vi "Table_Script.vi"() -> ()   [LabVIEW 2020]
uses:
  <userlib>/_OpenG.lib/array/array.llb/Index 1D Array Elements (String)__ogtk.vi
  <vilib>/regexp/Match Regular Expression.xnode
  <vilib>/addons/database/NI_Database_API.lvlib
panel:
  in  "Push Mind Script":string
  in  "Update Trigger":string
  in  "Insert Trigger":string
  in  "SELECT Into":string
  out "tables":string[](array[string])
  in  "HMI Script":string
  in  "PLC Tags":string
  in  "OPC Tag":bool
  in  "INSERTED":string
  in  "OPC Tags":string
  in  "Cluster":bool
  in  "Declare":string
  in  "Include Space":bool
  in  "Include Set Bracket":bool=TRUE
  in  "Script Column":string
  in  "Table List":i32[](listbox)
  # "Tag Name,Address,Data Type,Respect Data Type,Client Access,Scan Rate,Scaling,Raw Low,Raw High,Scaled Low,Scaled High,Scaled Data Type,Clamp Low,Clamp High,Eng Units,Description,Negate Value"
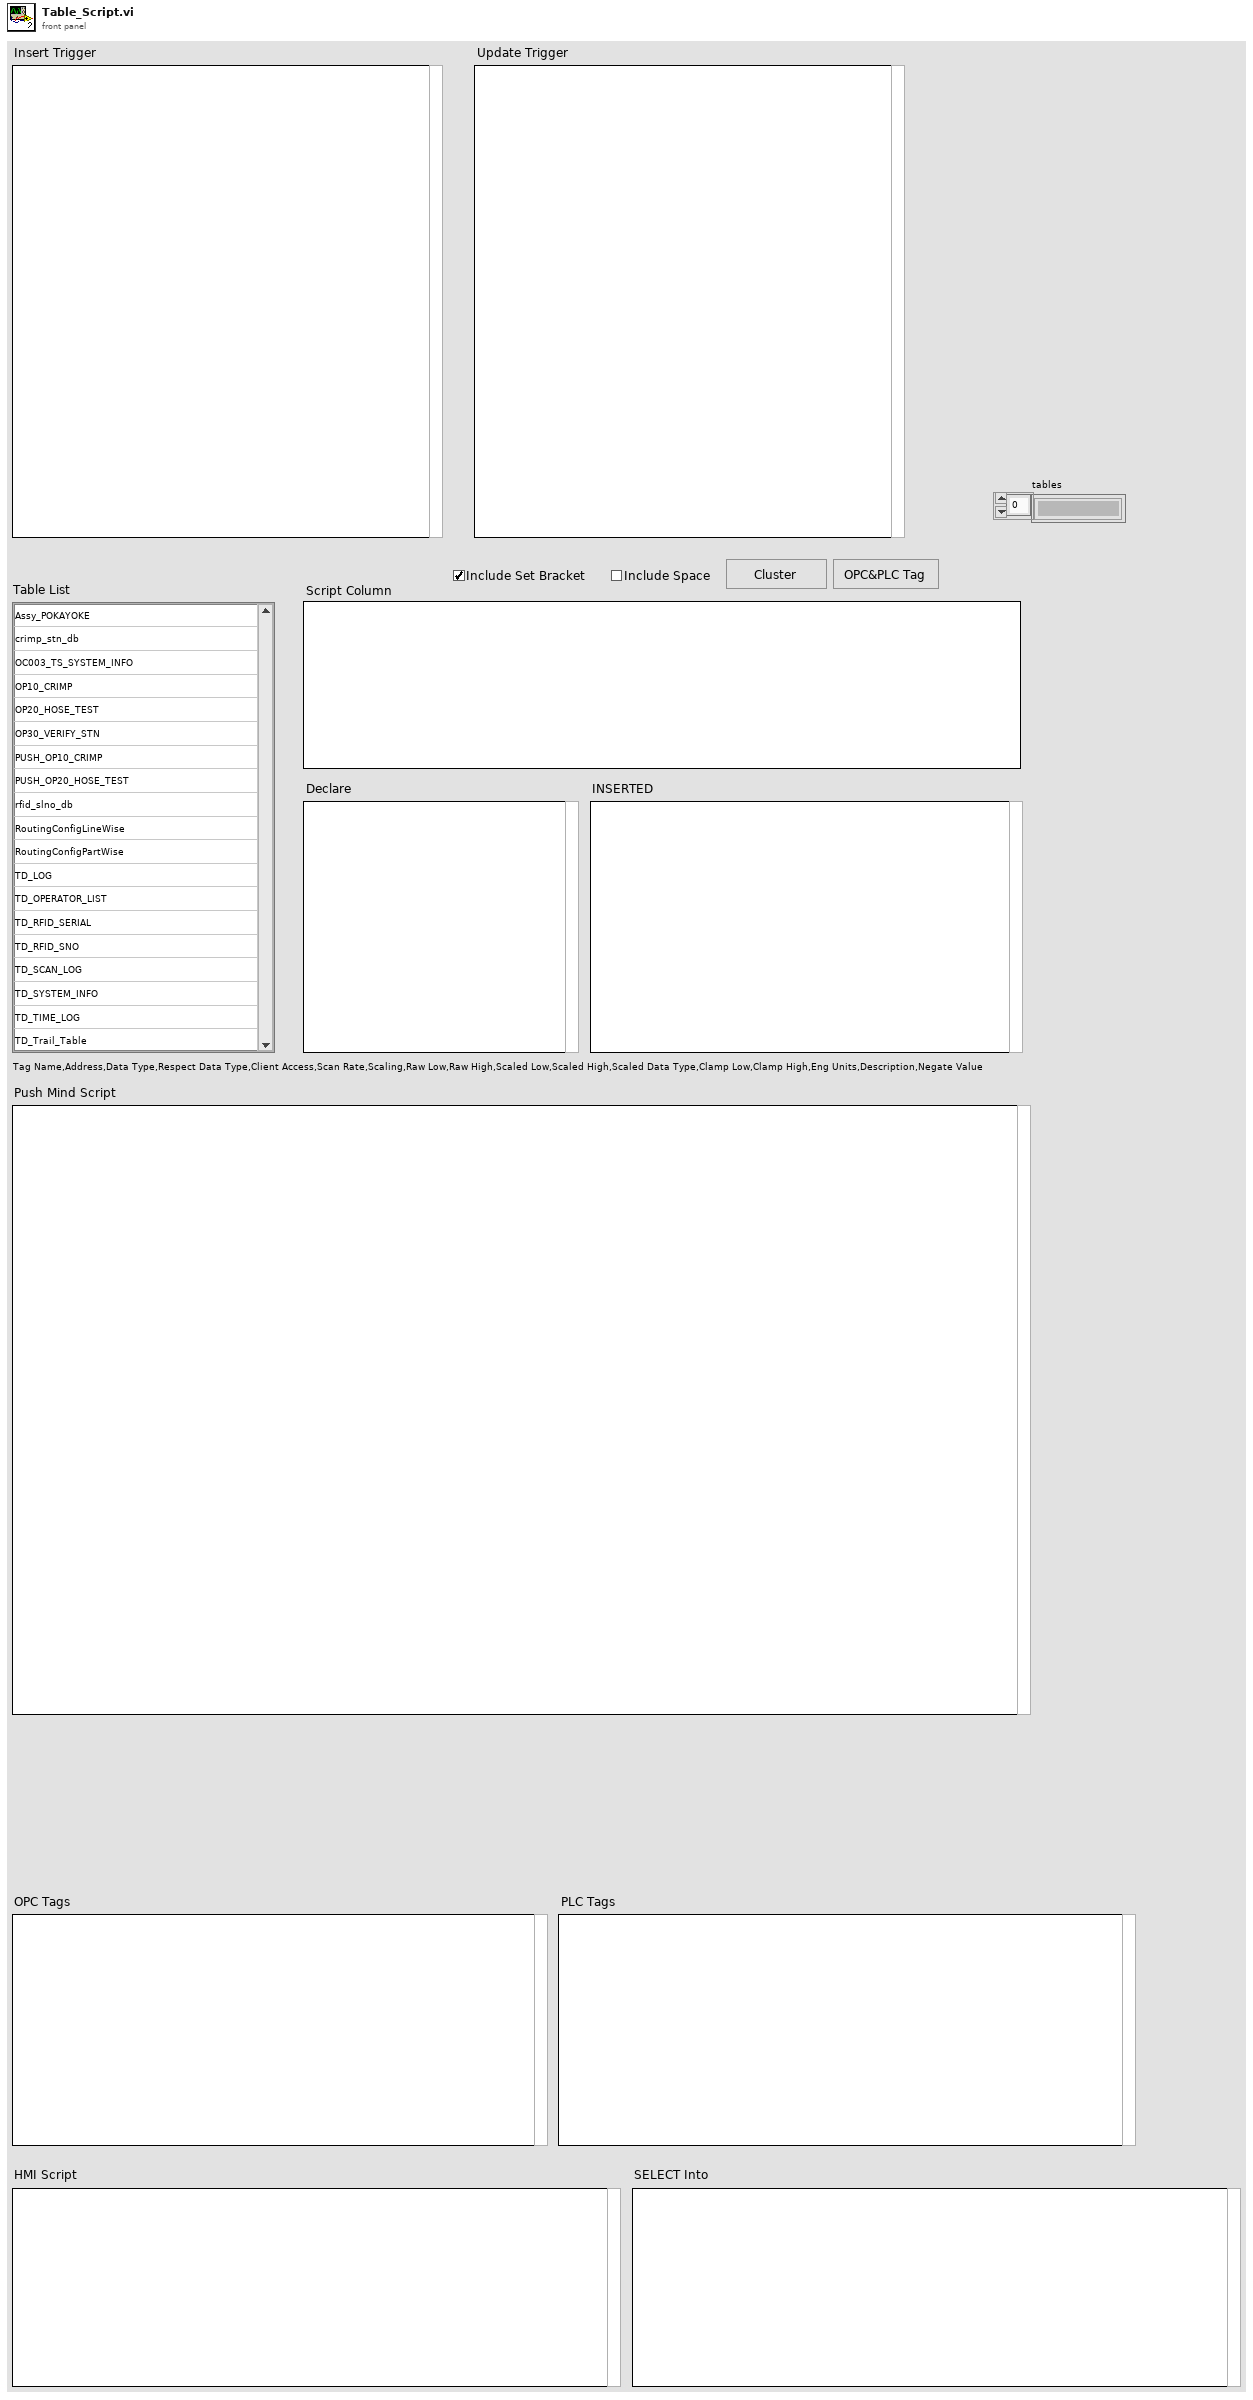
[diagram p1: front panel]
types:
  T1 = cluster{"Calibration":bool, "Settings":bool, "Script":bool, "Desktop Report":bool, "Help":bool}
  T2 = typedef "TD SQL.ctl" = cluster{"MS SQL Connection":T3, "UDL File":path, "Time":string, "DCODE":string, "WIP+1":i64, "MC No?":i32, "POKAYOKE?":bool, "Expected Result":string, "Result [Status]":string, "Clock":dbl, "RFID":string, "WIP Queue":refnum<queue>, "TS Parameter":T4, "Data_Queue":refnum<queue>[], "RFID Serial No.":string}
  T3 = typedef "NI_Database_API.lvlib/Conn ObjectReference.ctl" = refnum<k1>
  T4 = typedef "TS_Parameter.ctl" = cluster{"ProfitCenterCode":string, "LineCode":string, "WorkOrderNumber":string, "Model":string, "Model_with_Prefix":string, "VendorCode":string, "SetParameterDateCode":string, "PokaYoke":i32, "Target":i32, "Live_DateCode":string, "CustomerPartNumber":string, "Hand":string, "Ent_Stamp":timestamp, "STS_CD":dbl}
  T5 = typedef "NI_Database_API.lvlib/DB Tools DataTypes.ctl" = enum16{"String", "Long (I32)", "Single (SGL)", "Double (DBL)", "Date/Time", "Binary"}
  T6 = cluster{"name":string, "database data type":T5, "defined size":i32}[]
  T7 = cluster{"Data Path":path, "Calibration Path":path, "Settings Path":path, "Script Path":path, "DAQ Support":path, "Reporting Desktop":path, "Help":path}
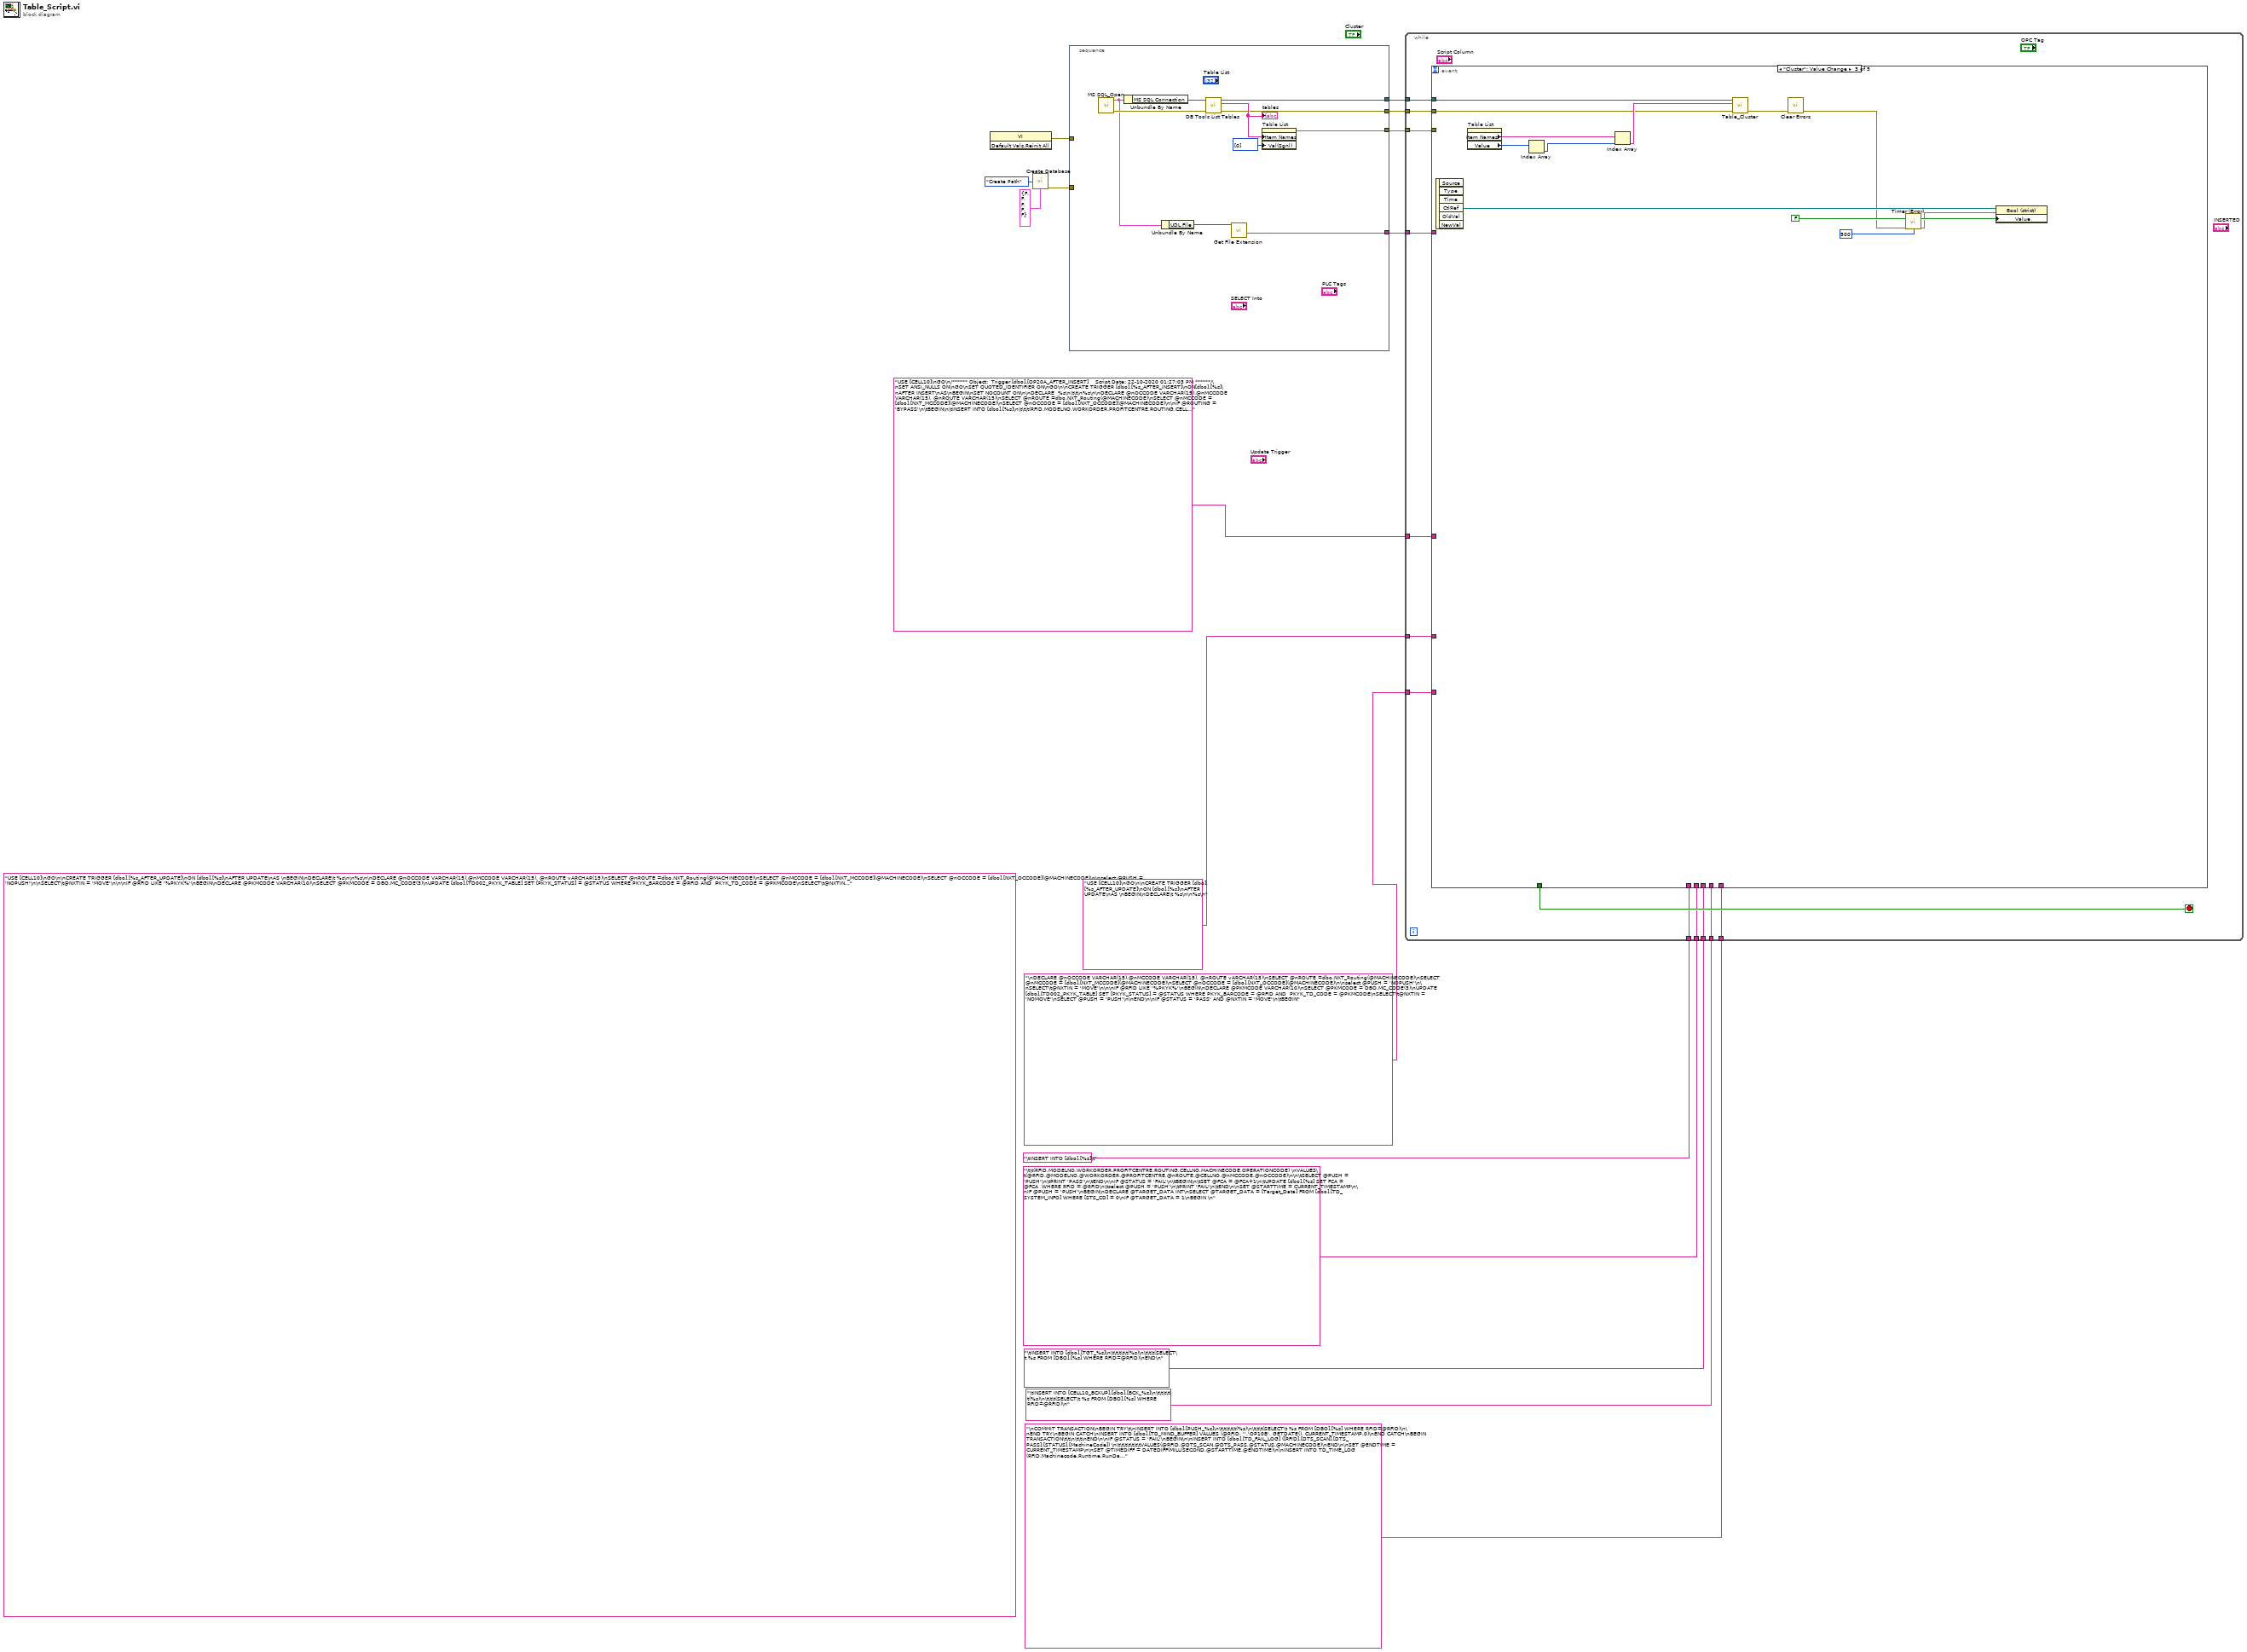
[diagram p0: block diagram]
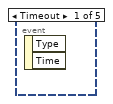
[diagram p2: hidden frame]
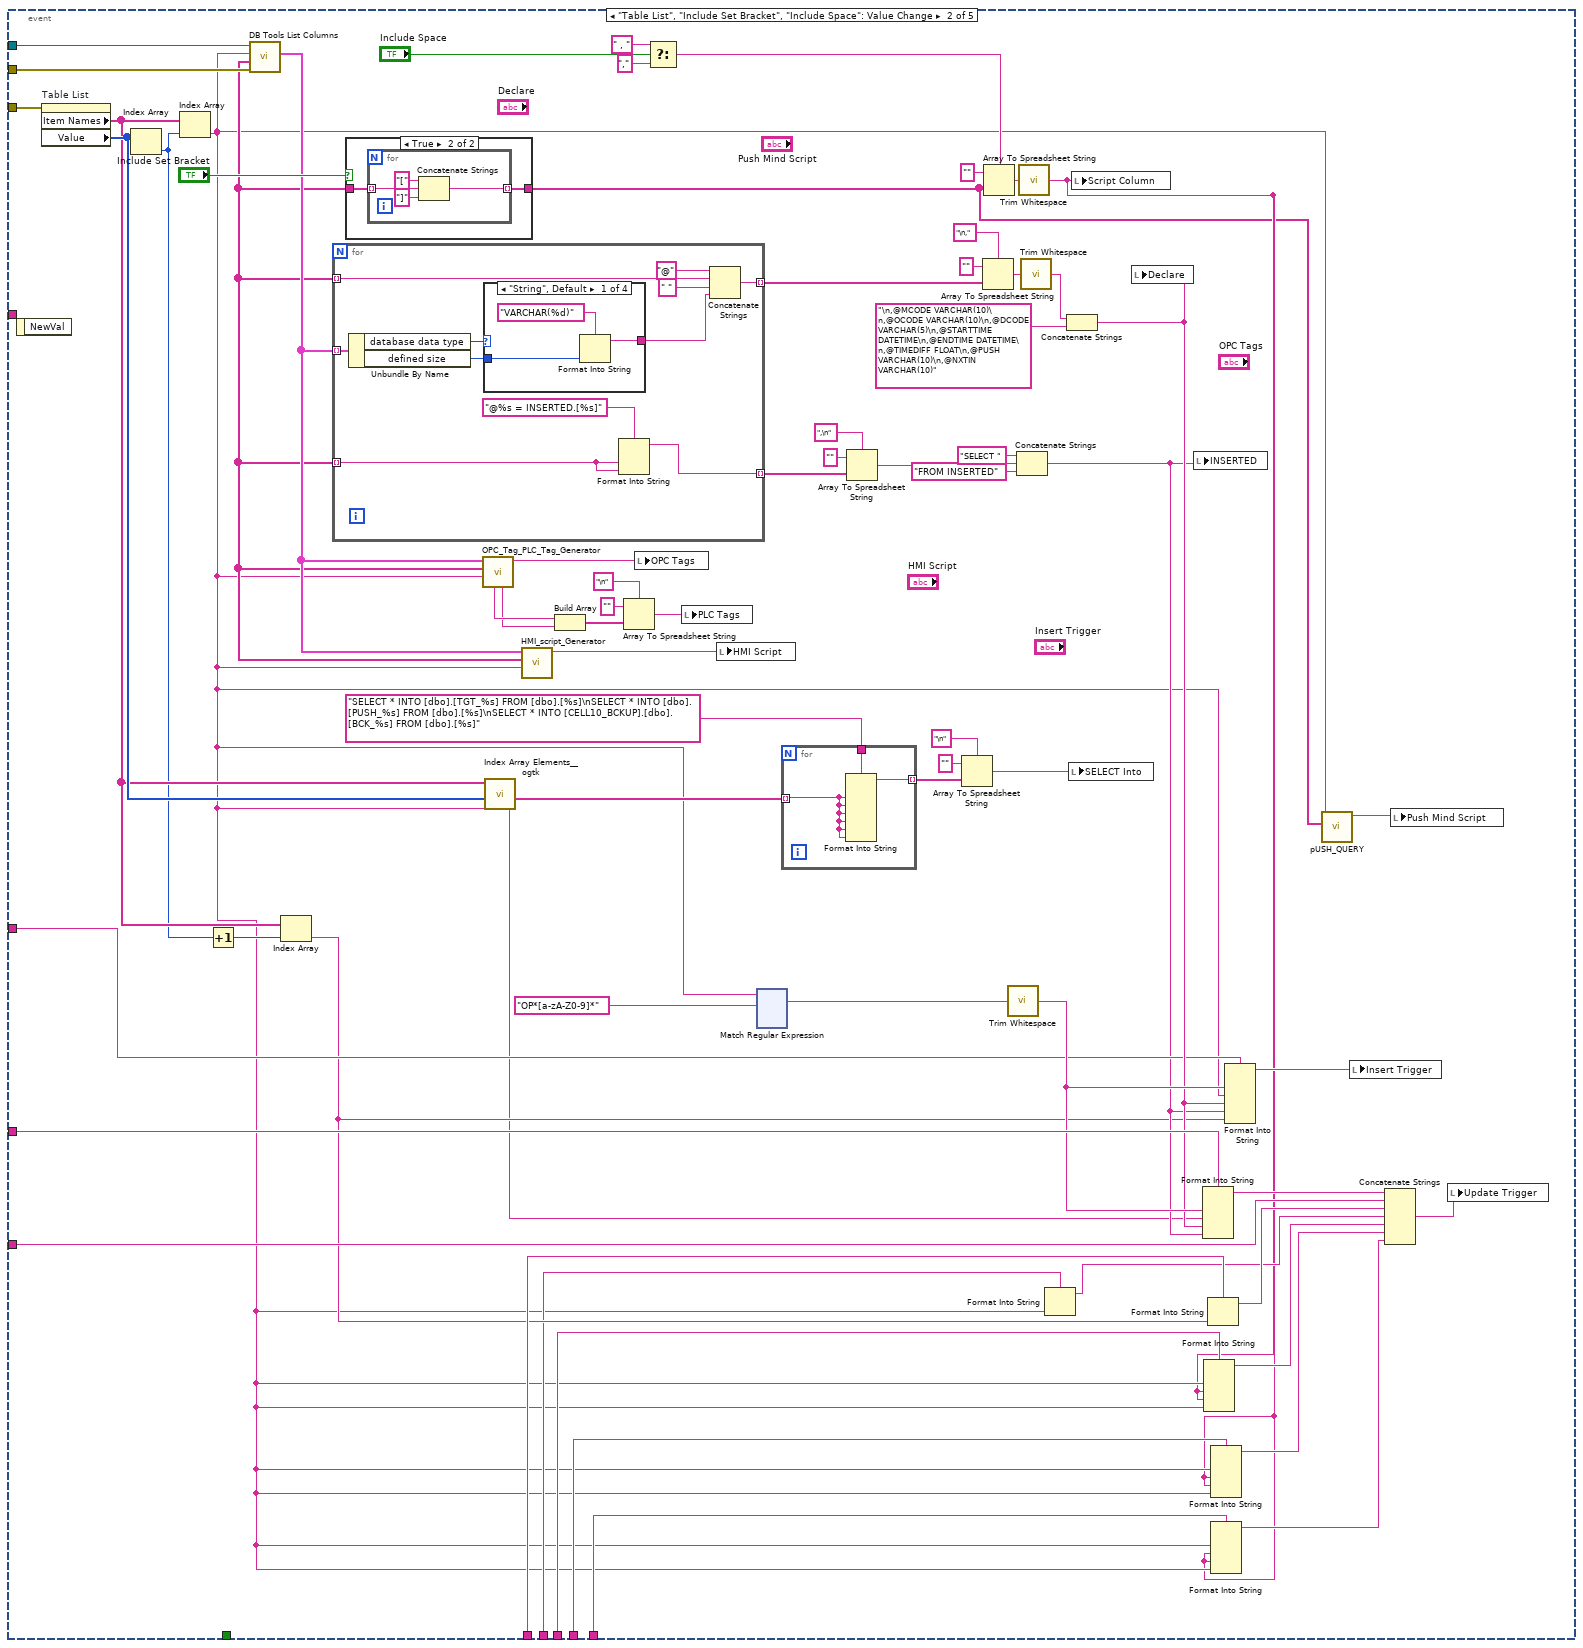
[diagram p3: hidden frame]
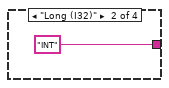
[diagram p4: hidden frame]
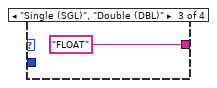
[diagram p5: hidden frame]
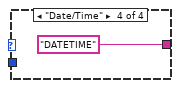
[diagram p6: hidden frame]
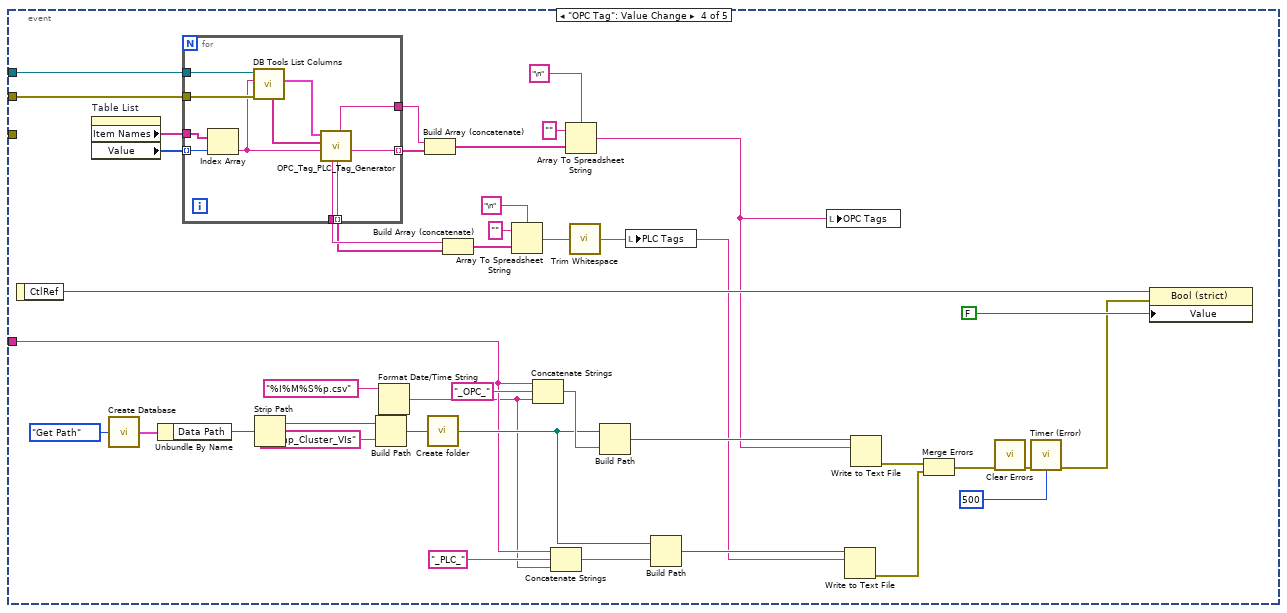
[diagram p8: hidden frame]
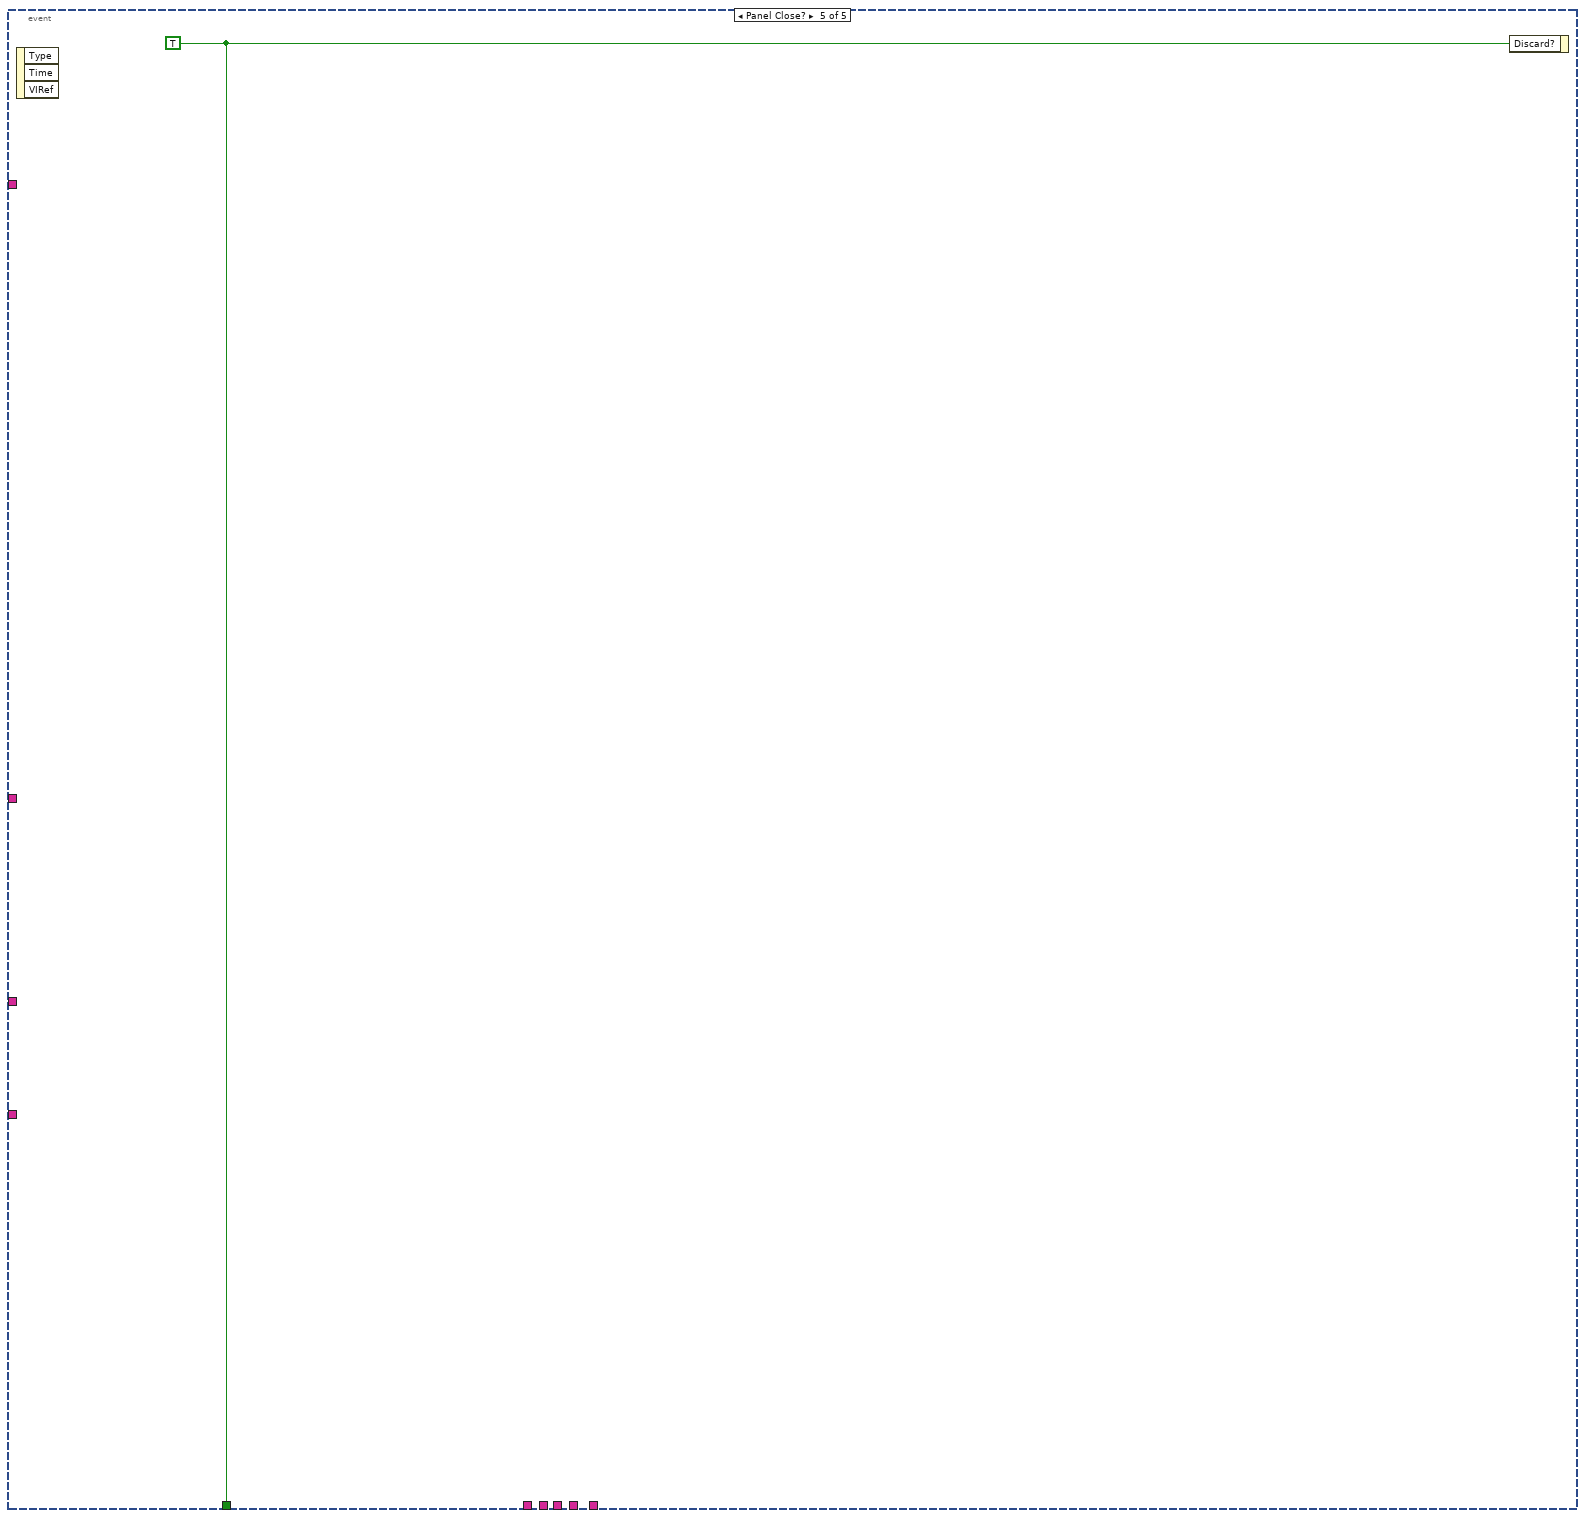
[diagram p9: hidden frame]
diagram:
  (unwired) "USE [CELL10]\nGO\n\nCREATE TRIGGER [dbo].[%s_AFTER_UPDATE]\nON [dbo].[%s]\nAFTER UPDATE\nAS \nBEGIN\nDECLARE\t %s\n\n%s\n\nDECLARE @nOCCODE VARCHAR(15),@nMCCODE VARCHAR(15), @nROUTE vARCHAR(15)\nSELECT @nROUTE =dbo.NXT_Routing(@MACHINECODE)\nSELECT @nMCCODE = [dbo].[NXT_MCCODE](@MACHINECODE)\nSELECT @nOCCODE = [dbo].[NXT_OCCODE](@MACHINECODE)\n\nselect @PUSH = 'NOPUSH'\n\nSELECT\t@NXTIN = 'MOVE'\n\n\nIF @RFID LIKE '%PKYK%'\nBEGIN\nDECLARE @PKMCODE VARCHAR(10)\nSELECT @PKMCODE = DBO.MC_CODE(3)\nUPDATE [dbo].[TD002_PKYK_TABLE] SET [PKYK_STATUS] = @STATUS WHERE PKYK_BARCODE = @RFID AND  PKYK_TD_CODE = @PKMCODE\nSELECT\t@NXTIN = 'NOMOVE'\nSELECT @PUSH = 'PUSH'\n\nEND\n\n\nIF @STATUS = 'PASS' AND @NXTIN = 'MOVE'\n\tBEGIN\n\tINSERT INTO [dbo].[%s]\t\n\t\t(RFID,MODELNO,WORKORDER,PROFITCENTRE,ROUTING,CELLNO,MACHINECODE,OPERATIONCODE) \nVALUES\t(@RFID,@MODELNO,@WORKORDER,@PROFITCENTRE,@nROUTE,@CELLNO,@nMCCODE,@nOCCODE)\n\n\tSELECT @PUSH = 'PUSH'\n\tPRINT 'PASS'\n\tEND\n\nIF @STATUS = 'FAIL'\n\tBEGIN\n\tSET @FCA = @FCA+1\n\tUPDATE [dbo].[%s] SET FCA = @FCA  WHERE RFID = @RFID\n\tselect @PUSH = 'PUSH'\n\tPRINT 'FAIL'\n\tEND\n\nSET @STARTTIME = CURRENT_TIMESTAMP\n\nIF @PUSH = 'PUSH'\nBEGIN\nDECLARE @TARGET_DATA INT\nSELECT @TARGET_DATA = [Target_Data] FROM [dbo].[TD_SYSTEM_INFO] WHERE [STS_CD] = 0\nIF @TARGET_DATA = 1\nBEGIN \n\tINSERT INTO [dbo].[TGT_OP20A_003_ACTUATOR_CIRCLIP_ASSY]\n\t\t\t\t\t([RFID],[DTS_SCAN],[DTS_PASS],[PUSHROD_HT_MIN],[PUSHROD_HT],[PUSHROD_HT_MAX],[CT],[STATUS],[FCS],[FCA],[ROUTING],[MODELNO],[WORKORDER],[CELLNO],[PROFITCENTRE],[MACHINECODE],[OPERATIONCODE],[RESERVED_11],[RESERVED_12],[RESERVED_13],[RESERVED_14],[RESERVED_15])\n\t\t\t(SELECT\t [RFID],[DTS_SCAN],[DTS_PASS],[PUSHROD_HT_MIN],[PUSHROD_HT],[PUSHROD_HT_MAX],[CT],[STATUS],[FCS],[FCA],[ROUTING],[MODELNO],[WORKORDER],[CELLNO],[PROFITCENTRE],[MACHINECODE],[OPERATIONCODE],[RESERVED_11],[RESERVED_12],[RESERVED_13],[RESERVED_14],[RESERVED_15] FROM [DBO].[OP20A_003_ACTUATOR_CIRCLIP_ASSY] WHERE RFID=@RFID)\n\nEND\n\n\tINSERT INTO [CELL10_BCKUP].[dbo].[BCK_OP20A_003_ACTUATOR_CIRCLIP_ASSY]\n\t\t\t\t\t([RFID],[DTS_SCAN],[DTS_PASS],[PUSHROD_HT_MIN],[PUSHROD_HT],[PUSHROD_HT_MAX],[CT],[STATUS],[FCS],[FCA],[ROUTING],[MODELNO],[WORKORDER],[CELLNO],[PROFITCENTRE],[MACHINECODE],[OPERATIONCODE],[RESERVED_11],[RESERVED_12],[RESERVED_13],[RESERVED_14],[RESERVED_15])\n\t\t\t(SELECT\t [RFID],[DTS_SCAN],[DTS_PASS],[PUSHROD_HT_MIN],[PUSHROD_HT],[PUSHROD_HT_MAX],[CT],[STATUS],[FCS],[FCA],[ROUTING],[MODELNO],[WORKORDER],[CELLNO],[PROFITCENTRE],[MACHINECODE],[OPERATIONCODE],[RESERVED_11],[RESERVED_12],[RESERVED_13],[RESERVED_14],[RESERVED_15] FROM [DBO].[OP20A_003_ACTUATOR_CIRCLIP_ASSY] WHERE RFID=@RFID)\n\nCOMMIT TRANSACTION\nBEGIN TRY\n\tINSERT INTO [dbo].[PUSH_OP20A_003_ACTUATOR_CIRCLIP_ASSY]\n\t\t\t\t\t([RFID],[DTS_SCAN],[DTS_PASS],[PUSHROD_HT_MIN],[PUSHROD_HT],[PUSHROD_HT_MAX],[CT],[STATUS],[FCS],[FCA],[ROUTING],[MODELNO],[WORKORDER],[CELLNO],[PROFITCENTRE],[MACHINECODE],[OPERATIONCODE],[RESERVED_11],[RESERVED_12],[RESERVED_13],[RESERVED_14],[RESERVED_15])\n\t\t\t(SELECT\t [RFID],[DTS_SCAN],[DTS_PASS],[PUSHROD_HT_MIN],[PUSHROD_HT],[PUSHROD_HT_MAX],[CT],[STATUS],[FCS],[FCA],[ROUTING],[MODELNO],[WORKORDER],[CELLNO],[PROFITCENTRE],[MACHINECODE],[OPERATIONCODE],[RESERVED_11],[RESERVED_12],[RESERVED_13],[RESERVED_14],[RESERVED_15] FROM [DBO].[OP20A_003_ACTUATOR_CIRCLIP_ASSY] WHERE RFID=@RFID)\n\nEND TRY\nBEGIN CATCH\nINSERT INTO [dbo].[TD_MIND_BUFFER] VALUES (@RFID, '','OP10B', GETDATE(), CURRENT_TIMESTAMP,0)\nEND CATCH\nBEGIN TRANSACTION\t\t\n\t\t\nEND\n\nIF @STATUS = 'FAIL'\nBEGIN\n\nINSERT INTO [dbo].[TD_FAIL_LOG] ([RFID],[DTS_SCAN],[DTS_PASS],[STATUS],[MachineCode]) \n\t\t\t\t\t\t\tVALUES(@RFID,@DTS_SCAN,@DTS_PASS,@STATUS,@MACHINECODE)\nEND\n\n\n\nSET @ENDTIME = CURRENT_TIMESTAMP\n\nSET @TIMEDIFF = DATEDIFF(MILLISECOND,@STARTTIME,@ENDTIME)\n\nINSERT INTO TD_TIME_LOG (RFID,Machinecode,Runtime,RunDate) values(@RFID,@MACHINECODE,@TIMEDIFF,CURRENT_TIMESTAMP)\n\nEND\n" ("delimiter (Tab)")
  n1 = invoke class="VI" method="Default Vals.Reinit All"() -> (error out=w10:errorcluster)  [unwired: 3 in, 2 out]
  n2 = call <userlib>:"Create Database.vi"("Get/Create"=enum16{"Get Path", "Create Path"}."Create Path", "Create Folder"=T1 {"Calibration"=FALSE, "Settings"=FALSE, "Script"=FALSE, "Desktop Report"=FALSE, "Help"=FALSE}) -> ("error out"=w12:errorcluster)  [unwired: 12 in, 1 out]
  n3 = stacked-sequence {
    tunnel: [w23] -> w16
    tunnel: [w22] -> w15
    tunnel: [w21] -> w14
    tunnel: w12 -> [_]
    tunnel: w10 -> [_]
    tunnel: [w17] -> w9
    frame #0 {
      n4 = call "MS SQL_Open.vi"() -> ("error out"=w25:errorcluster, "Ref Out"=w19:T2)  [unwired: 9 in, 1 out]
      n5 = Unbundle By Name(w19) -> ("MS SQL Connection"=w26:T3)
      n6 = Unbundle By Name(w19) -> ("UDL File"=w18:path)
      n7 = call <vilib>:"DB Tools List Tables.vi"("error in (no error)"=w25, "connection reference"=w26) -> ("error out"=w21:errorcluster, "tables"=w24:string[], "connection reference out"=w22:T3)  [unwired: 3 in]
      "tables" <- w24
      n8 = call <vilib>:"Get File Extension.vi"("file"=w18) -> ("filename without extension"=w17:string)  [unwired: 6 in, 4 out]
      n9 = property on="Table List" class="LstBox (strict)"("Item Names"=w24, "Val(Sgnl)"=i32[] [0] ("Value (Signaling)")) -> (error out=w23:errorcluster)  [unwired: 2 in, 1 out]
    }
  }
  n10 = while {
    tunnel: w16 -> [w38]
    tunnel: w15 -> [w37]
    tunnel: w14 -> [w36]
    tunnel: w9 -> [w35]
    tunnel: "USE [CELL10]\nGO\n/****** Object:  Trigger [dbo].[OP20A_AFTER_INSERT]    Script Date: 22-10-2020 01:27:03 PM ******/\nSET ANSI_NULLS ON\nGO\nSET QUOTED_IDENTIFIER ON\nGO\n\nCREATE TRIGGER [dbo].[%s_AFTER_INSERT]\nON[dbo].[%s]\nAFTER INSERT\nAS\nBEGIN\nSET NOCOUNT ON\n\nDECLARE  %s\n\t\t\n%s\n\nDECLARE @nOCCODE VARCHAR(15),@nMCCODE VARCHAR(15), @nROUTE VARCHAR(15)\nSELECT @nROUTE =dbo.NXT_Routing(@MACHINECODE)\nSELECT @nMCCODE = [dbo].[NXT_MCCODE](@MACHINECODE)\nSELECT @nOCCODE = [dbo].[NXT_OCCODE](@MACHINECODE)\n\nIF @ROUTING = 'BYPASS'\n\tBEGIN\n\tINSERT INTO [dbo].[%s]\n\t\t\t(RFID,MODELNO,WORKORDER,PROFITCENTRE,ROUTING,CELLNO,MACHINECODE,OPERATIONCODE) \n\tVALUES\t(@RFID,@MODELNO,@WORKORDER,@PROFITCENTRE,@nROUTE,@CELLNO,@nMCCODE,@nOCCODE)\n\tEND\n\nend\n\n" ("delimiter (Tab)") -> [w34]
    tunnel: "USE [CELL10]\nGO\n\nCREATE TRIGGER [dbo].[%s_AFTER_UPDATE]\nON [dbo].[%s]\nAFTER UPDATE\nAS \nBEGIN\nDECLARE\t %s\n\n%s\n" -> [w33]
    tunnel: "\nDECLARE @nOCCODE VARCHAR(15),@nMCCODE VARCHAR(15), @nROUTE vARCHAR(15)\nSELECT @nROUTE =dbo.NXT_Routing(@MACHINECODE)\nSELECT @nMCCODE = [dbo].[NXT_MCCODE](@MACHINECODE)\nSELECT @nOCCODE = [dbo].[NXT_OCCODE](@MACHINECODE)\n\nselect @PUSH = 'NOPUSH'\n\nSELECT\t@NXTIN = 'MOVE'\n\n\nIF @RFID LIKE '%PKYK%'\nBEGIN\nDECLARE @PKMCODE VARCHAR(10)\nSELECT @PKMCODE = DBO.MC_CODE(3)\nUPDATE [dbo].[TD002_PKYK_TABLE] SET [PKYK_STATUS] = @STATUS WHERE PKYK_BARCODE = @RFID AND  PKYK_TD_CODE = @PKMCODE\nSELECT\t@NXTIN = 'NOMOVE'\nSELECT @PUSH = 'PUSH'\n\nEND\n\nIF @STATUS = 'PASS' AND @NXTIN = 'MOVE'\n\tBEGIN" -> [w32]
    tunnel: "\tINSERT INTO [dbo].[%s]\t" -> [w31]
    tunnel: "\t\t(RFID,MODELNO,WORKORDER,PROFITCENTRE,ROUTING,CELLNO,MACHINECODE,OPERATIONCODE) \nVALUES\t(@RFID,@MODELNO,@WORKORDER,@PROFITCENTRE,@nROUTE,@CELLNO,@nMCCODE,@nOCCODE)\n\n\tSELECT @PUSH = 'PUSH'\n\tPRINT 'PASS'\n\tEND\n\nIF @STATUS = 'FAIL'\n\tBEGIN\n\tSET @FCA = @FCA+1\n\tUPDATE [dbo].[%s] SET FCA = @FCA  WHERE RFID = @RFID\n\tselect @PUSH = 'PUSH'\n\tPRINT 'FAIL'\n\tEND\n\nSET @STARTTIME = CURRENT_TIMESTAMP\n\nIF @PUSH = 'PUSH'\nBEGIN\nDECLARE @TARGET_DATA INT\nSELECT @TARGET_DATA = [Target_Data] FROM [dbo].[TD_SYSTEM_INFO] WHERE [STS_CD] = 0\nIF @TARGET_DATA = 1\nBEGIN \n" -> [w30]
    tunnel: "\tINSERT INTO [dbo].[TGT_%s]\n\t\t\t\t\t(%s)\n\t\t\t(SELECT\t %s FROM [DBO].[%s] WHERE RFID=@RFID)\nEND\n" -> [w29]
    tunnel: "\tINSERT INTO [CELL10_BCKUP].[dbo].[BCK_%s]\n\t\t\t\t\t(%s)\n\t\t\t(SELECT\t %s FROM [DBO].[%s] WHERE RFID=@RFID)\n" -> [w28]
    tunnel: "\nCOMMIT TRANSACTION\nBEGIN TRY\t\nINSERT INTO [dbo].[PUSH_%s]\n\t\t\t\t\t(%s)\n\t\t\t(SELECT\t %s FROM [DBO].[%s] WHERE RFID=@RFID)\n\nEND TRY\nBEGIN CATCH\nINSERT INTO [dbo].[TD_MIND_BUFFER] VALUES (@RFID, '','OP10B', GETDATE(), CURRENT_TIMESTAMP,0)\nEND CATCH\nBEGIN TRANSACTION\t\t\n\t\t\nEND\n\nIF @STATUS = 'FAIL'\nBEGIN\n\nINSERT INTO [dbo].[TD_FAIL_LOG] ([RFID],[DTS_SCAN],[DTS_PASS],[STATUS],[MachineCode]) \n\t\t\t\t\t\t\tVALUES(@RFID,@DTS_SCAN,@DTS_PASS,@STATUS,@MACHINECODE)\nEND\n\nSET @ENDTIME = CURRENT_TIMESTAMP\n\nSET @TIMEDIFF = DATEDIFF(MILLISECOND,@STARTTIME,@ENDTIME)\n\nINSERT INTO TD_TIME_LOG (RFID,Machinecode,Runtime,RunDate) values(@RFID,@MACHINECODE,@TIMEDIFF,CURRENT_TIMESTAMP)\n\nEND\n" -> [w27]
    stop <- w39 stop-if-true
    n11 = event shown="[2] \"Cluster\": Value Change" {
      selector: _ -> [_ _ _ _ _]
      dyn-events: _ -> [_ _ _ _ _]
      timeout: _ -> [_ _ _ _ _]
      tunnel: [_ _ _ _ w313] -> w39
      tunnel: w38 -> [_ w107 _ _ _]
      tunnel: w37 -> [_ w106 w257 w285 _]
      tunnel: w36 -> [_ w105 w256 w284 _]
      tunnel: w35 -> [_ _ _ w269 _]
      tunnel: w34 -> [_ w58 _ _ _]
      tunnel: w33 -> [_ w62 _ _ _]
      tunnel: w32 -> [_ w55 _ _ _]
      tunnel: w31 -> [_ w54 _ _ _]
      tunnel: w30 -> [_ w45 _ _ _]
      tunnel: w29 -> [_ w51 _ _ _]
      tunnel: w28 -> [_ w49 _ _ _]
      tunnel: w27 -> [_ w48 _ _ _]
      event Timeout {
        n12 = event-data() -> ()  [unwired: 1 in, 2 out]
      }
      event "Table List", "Include Set Bracket", "Include Space": Value Change {
        n13 = event-data() -> ()  [unwired: 1 in, 1 out]
        n14 = property on="Table List" class="LstBox (strict)"(error in=w107) -> ("Item Names"=w65:string[], "Value"=w74:i32[])  [unwired: 1 in, 2 out]
        n15 = Index Array(array=w74) -> (element=w64:i32)  [unwired: 1 in]
        n16 = Index Array(array=w65, index=w64) -> (element=w43:string)
        n17 = Increment(x=w64) -> (x+1=w63:i32)
        n18 = call <vilib>:"DB Tools List Columns.vi"("error in (no error)"=w105, "table"=w43, "connection reference"=w106) -> ("columns"=w77:string[], "column information"=w78:T6)  [unwired: 1 in, 2 out]
        n19 = Index Array(array=w65, index=w63) -> (element=w53:string)
        n20 = for {
          tunnel: w77 -> [w225] mode=indexing
          tunnel: [w234] -> w96 mode=indexing
          tunnel: w78 -> [w233] mode=indexing
          tunnel: w77 -> [w227] mode=indexing
          tunnel: [w226] -> w91 mode=indexing
          n21 = Unbundle By Name(w233) -> ("database data type"=w229:T5, "defined size"=w232:i32)
          n22 = case shown="\"String\", Default" w229 {
            tunnel: w232 -> [w237 _ _ _]
            tunnel: [w236 "INT" "FLOAT" "DATETIME"] -> w230
            frame "String", Default {
              n23 = Format Into String(format string="VARCHAR(%d)" ("string"), w237) -> (resulting string=w236:string)  [unwired: 2 in, 1 out]
            }
            frame "Long (I32)" {
            }
            frame "Single (SGL)", "Double (DBL)" {
            }
            frame "Date/Time" {
            }
          }
          n24 = Format Into String(format string="@%s = INSERTED.[%s]", w227, w227) -> (resulting string=w226:string)  [unwired: 2 in, 1 out]
          n25 = Concatenate Strings("@" ("string"), w225, " " ("string"), w230) -> (w234:string)
        }
        n26 = case shown="True" "Include Set Bracket" {
          tunnel: w77 -> [w242 w244]
          tunnel: [w242 w243] -> w41
          frame False {
          }
          frame True {
            n27 = for {
              tunnel: w244 -> [w248] mode=indexing
              tunnel: [w245] -> w243 mode=indexing
              n28 = Concatenate Strings("[" ("string"), w248, "]" ("string")) -> (w245:string)
            }
          }
        }
        n29 = call "OPC_Tag_PLC_Tag_Generator.vi"("Table Name"=w43, "Columns"=w77, "column information"=w78) -> ("OPC Tags"=w94:string, "PLC Tag only"=w80:string, "PLC Header"=w81:string)  [unwired: 4 in, 2 out]
        n30 = call-poly <userlib>:"Index Array Elements__ogtk.vi"("indices"=w74, "array"=w65) -> ("elements"=w73:string[])  [unwired: 9 in]
        n31 = call "HMI_script_Generator.vi"("Table Name"=w43, "Columns"=w77, "column information"=w78) -> ("HMI Script"=w76:string)  [unwired: 8 in]
        n32 = Build Array(w81, w80) -> (w82:string[])
        n33 = Array To Spreadsheet String(delimiter (Tab)="\n", array=w82, 3:"" ("format string")) -> (spreadsheet string=w79:string)
        n34 = local write "OPC Tags"(w94) -> ()
        n35 = Select(t=" , " ("delimiter (Tab)"), s="Include Space", f=",") -> (s? t:f=w98:string)
        n36 = local write "PLC Tags"(w79) -> ()
        n37 = local write "HMI Script"(w76) -> ()
        n38 = xnode "Match Regular Expression"("input string"=w43, "regular expression"="OP*[a-zA-Z0-9]*" ("String")) -> ("whole match"=w68:string)  [unwired: 4 in, 4 out]
        n39 = for {
          tunnel: "SELECT * INTO [dbo].[TGT_%s] FROM [dbo].[%s]\nSELECT * INTO [dbo].[PUSH_%s] FROM [dbo].[%s]\nSELECT * INTO [CELL10_BCKUP].[dbo].[BCK_%s] FROM [dbo].[%s]" ("delimiter (Tab)") -> [w224]
          tunnel: w73 -> [w223] mode=indexing
          tunnel: [w222] -> w70 mode=indexing
          n40 = Format Into String(format string=w224, w223, w223, w223, w223, w223, w223) -> (resulting string=w222:string)  [unwired: 2 in, 1 out]
        }
        n41 = Array To Spreadsheet String(delimiter (Tab)=",\n", array=w91, 3:"" ("format string")) -> (spreadsheet string=w90:string)
        n42 = Array To Spreadsheet String(delimiter (Tab)="\n", array=w70, 3:"" ("format string")) -> (spreadsheet string=w69:string)
        n43 = Array To Spreadsheet String(delimiter (Tab)="\n,", array=w96, 3:"" ("format string")) -> (spreadsheet string=w87:string)
        n44 = Array To Spreadsheet String(delimiter (Tab)=w98, array=w41, 3:"" ("format string")) -> (spreadsheet string=w103:string)
        n45 = call <vilib>:"Trim Whitespace.vi"("string"=w68) -> ("trimmed string"=w61:string)  [unwired: 1 in]
        n46 = Concatenate Strings("SELECT " ("string"), w90, "FROM INSERTED" ("string")) -> (w57:string)
        n47 = call <vilib>:"Trim Whitespace.vi"("string"=w103) -> ("trimmed string"=w42:string)  [unwired: 1 in]
        n48 = call <vilib>:"Trim Whitespace.vi"("string"=w87) -> ("trimmed string"=w85:string)  [unwired: 1 in]
        n49 = Format Into String(format string=w45, w43) -> (resulting string=w44:string)  [unwired: 2 in, 1 out]
        n50 = Concatenate Strings(w85, "\n,@MCODE VARCHAR(10)\n,@OCODE VARCHAR(10)\n,@DCODE VARCHAR(5)\n,@STARTTIME DATETIME\n,@ENDTIME DATETIME\n,@TIMEDIFF FLOAT\n,@PUSH VARCHAR(10)\n,@NXTIN VARCHAR(10)" ("format string")) -> (w59:string)
        n51 = local write "SELECT Into"(w69) -> ()
        n52 = local write "Script Column"(w42) -> ()
        n53 = local write "Declare"(w59) -> ()
        n54 = local write "INSERTED"(w57) -> ()
        n55 = Format Into String(format string=w62, w61, w43, w59, w57) -> (resulting string=w60:string)  [unwired: 2 in, 1 out]
        n56 = Format Into String(format string=w51, w43, w42, w42, w43) -> (resulting string=w50:string)  [unwired: 2 in, 1 out]
        n57 = Format Into String(format string=w54, w53) -> (resulting string=w52:string)  [unwired: 2 in, 1 out]
        n58 = Format Into String(format string=w49, w43, w42, w42, w43) -> (resulting string=w47:string)  [unwired: 2 in, 1 out]
        n59 = Format Into String(format string=w48, w43, w42, w42, w43) -> (resulting string=w46:string)  [unwired: 2 in, 1 out]
        n60 = Format Into String(format string=w58, w61, w43, w59, w57, w53) -> (resulting string=w66:string)  [unwired: 2 in, 1 out]
        n61 = call "pUSH_QUERY.vi"("columns"=w41, "Table Name"=w43) -> ("resulting string"=w40:string)  [unwired: 9 in]
        n62 = local write "Insert Trigger"(w66) -> ()
        n63 = Concatenate Strings(w60, w55, w52, w44, w50, w47, w46) -> (w56:string)
        n64 = local write "Push Mind Script"(w40) -> ()
        n65 = local write "Update Trigger"(w56) -> ()
      }
      event "Cluster": Value Change {
        n66 = event-data() -> ("CtlRef"=w255:refnum<vi>)  [unwired: 1 in, 5 out]
        n67 = property on="Table List" class="LstBox (strict)"() -> ("Item Names"=w260:string[], "Value"=w258:i32[])  [unwired: 2 in, 2 out]
        n68 = Index Array(array=w258) -> (element=w249:i32)  [unwired: 1 in]
        n69 = Index Array(array=w260, index=w249) -> (element=w259:string)
        n70 = call "Table_Cluster.vi"("error in (no error)"=w256, "Table name"=w259, "Refnum in"=w257) -> ("error out"=w253:errorcluster)  [unwired: 8 in]
        n71 = call <vilib>:"Clear Errors.vi"("error in (no error)"=w253) -> ("error out"=w251:errorcluster)  [unwired: 5 in, 1 out]
        n72 = call <userlib>:"Timer (Error).vi"("error in (no error)"=w251, "milliseconds to wait"=u32 500) -> ("error out"=w250:errorcluster)  [unwired: 13 in]
        n73 = property class="Bool (strict)"(reference=w255, error in=w250, "Value"=FALSE) -> ()  [unwired: 2 out]
      }
      event "OPC Tag": Value Change {
        n74 = event-data() -> ("CtlRef"=w301:refnum<vi>)  [unwired: 1 in]
        n75 = property on="Table List" class="LstBox (strict)"() -> ("Item Names"=w282:string[], "Value"=w283:i32[])  [unwired: 2 in, 2 out]
        n76 = call <userlib>:"Create Database.vi"("Get/Create"=enum16{"Get Path", "Create Path"}."Get Path") -> ("Path Out"=w298:T7)  [unwired: 13 in, 1 out]
        n77 = Unbundle By Name(w298) -> ("Data Path"=w297:path)
        n78 = for {
          tunnel: w285 -> [w310]
          tunnel: w284 -> [w309]
          tunnel: w283 -> [w307] mode=indexing
          tunnel: w282 -> [w308]
          tunnel: [w305] -> w278 mode=indexing
          tunnel: [w304] -> w277
          tunnel: [w303] -> w272
          tunnel: [w302] -> w271 mode=indexing
          n79 = Index Array(array=w308, index=w307) -> (element=w306:string)
          n80 = call <vilib>:"DB Tools List Columns.vi"("error in (no error)"=w309, "table"=w306, "connection reference"=w310) -> ("columns"=w312:string[], "column information"=w311:T6)  [unwired: 1 in, 2 out]
          n81 = call "OPC_Tag_PLC_Tag_Generator.vi"("Table Name"=w306, "Columns"=w312, "column information"=w311) -> ("OPC Tag only"=w305:string, "PLC Tag only"=w302:string, "Header"=w304:string, "PLC Header"=w303:string)  [unwired: 4 in, 1 out]
        }
        n82 = Strip Path(path=w297) -> (stripped path=w296:path)  [unwired: 1 out]
        n83 = Build Path(base path=w296, name or relative path="Temp_Cluster_VIs") -> (appended path=w294:path)
        n84 = Format Date/Time String(time format string (%c)="%I%M%S%p.csv") -> (date/time string=w267:string)  [unwired: 2 in]
        n85 = Build Array (concatenate)(w277, w278) -> (w279:string[])
        n86 = call <userlib>:"Create folder.vi"("Path In"=w294) -> ("Path out"=w270:path)  [unwired: 14 in]
        n87 = Build Array (concatenate)(w272, w271) -> (w275:string[])
        n88 = Array To Spreadsheet String(delimiter (Tab)="\n", array=w275, 3:"" ("format string")) -> (spreadsheet string=w264:string)
        n89 = Concatenate Strings(w269, "_OPC_" ("string"), w267) -> (w291:string)
        n90 = Concatenate Strings(w269, "_PLC_" ("string"), w267) -> (w266:string)
        n91 = Array To Spreadsheet String(delimiter (Tab)="\n", array=w279, 3:"" ("format string")) -> (spreadsheet string=w276:string)
        n92 = call <vilib>:"Trim Whitespace.vi"("string"=w264) -> ("trimmed string"=w261:string)  [unwired: 1 in]
        n93 = Build Path(base path=w270, name or relative path=w291) -> (appended path=w290:path)
        n94 = local write "PLC Tags"(w261) -> ()
        n95 = Build Path(base path=w270, name or relative path=w266) -> (appended path=w265:path)
        n96 = local write "OPC Tags"(w276) -> ()
        n97 = Write to Text File(file (use dialog)=w265, text=w261) -> (error out=w262:errorcluster)  [unwired: 2 in, 2 out]
        n98 = Write to Text File(file (use dialog)=w290, text=w276) -> (error out=w289:errorcluster)  [unwired: 2 in, 2 out]
        n99 = Merge Errors(w289, w262) -> (w263:errorcluster)
        n100 = call <vilib>:"Clear Errors.vi"("error in (no error)"=w263) -> ("error out"=w288:errorcluster)  [unwired: 5 in, 1 out]
        n101 = call <userlib>:"Timer (Error).vi"("error in (no error)"=w288, "milliseconds to wait"=u32 500) -> ("error out"=w287:errorcluster)  [unwired: 13 in]
        n102 = property class="Bool (strict)"(reference=w301, error in=w287, "Value"=FALSE) -> ()  [unwired: 2 out]
      }
      event Panel Close? {
        w313 = TRUE ("Discard?")
        n103 = event-data() -> ()  [unwired: 1 in, 3 out]
        n104 = event-data("Discard?"=w313) -> ()  [unwired: 1 in, 1 out]
      }
    }
  }
